vi "beautifulVI.vi"() -> ()   [LabVIEW 2019]
panel:
  in  "Numeric 2":dbl
  out "Numeric":dbl
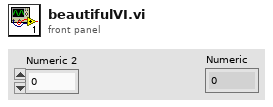
[diagram p1: front panel]
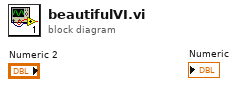
[diagram p0: block diagram]
diagram:
